vi "lijnvolgen.vi"() -> ()   [LabVIEW 2019]
uses:
  <vilib>/myRIO/Common/Instrument Driver Framework/Utilities/typedefs/Analog Scaling Constants.ctl
  <vilib>/myRIO/Common/Instrument Driver Framework/Utilities/typedefs/Analog Scaling Constants List.ctl
  <vilib>/myRIO/Common/Instrument Driver Framework/myRIO v1.0/AO/typedefs/AO Channels Enum.ctl
  <vilib>/myRIO/Common/Instrument Driver Framework/myRIO v1.0/AO/typedefs/AO Channels List.ctl
  <vilib>/myRIO/Common/Instrument Driver Framework/Utilities/typedefs/Generic FPGA Reference.ctl
  <vilib>/myRIO/Common/Instrument Driver Framework/Utilities/typedefs/myRIO v1.0 Reference.ctl
  <vilib>/myRIO/Common/Instrument Driver Framework/Utilities/typedefs/Hardware Version Enum.ctl
  <vilib>/myRIO/Common/Instrument Driver Framework/Utilities/typedefs/myRIO Generic Hardware Reference.ctl
  <vilib>/myRIO/Instrument Drivers/Onboard IO/AO/typedefs/AO Reference.ctl
  <vilib>/myRIO/Instrument Drivers/Onboard IO/AO/AO.lvlib
  <vilib>/myRIO/Instrument Drivers/Onboard IO/AO/vis/Write.vi
  <vilib>/userDefined/High Color/nirio_resource_hc.ctl
  <vilib>/myRIO/Common/Instrument Driver Framework/myRIO v1.0/AO/vis/myRIO v1.1 Open AO.vi
  <vilib>/myRIO/Instrument Drivers/Onboard IO/AO/vis/myRIO AO Open.xnode
  <vilib>/myRIO/Common/Instrument Driver Framework/Utilities/vis/Is FPGA Ref Available.vi
  <vilib>/myRIO/Express VI/Onboard IO/AO/AO Express VI.xnode
  <vilib>/myRIO/Common/Instrument Driver Framework/myRIO v1.0/AI/typedefs/AI Channels Enum.ctl
  <vilib>/myRIO/Common/Instrument Driver Framework/myRIO v1.0/AI/typedefs/AI Channels List.ctl
  <vilib>/myRIO/Instrument Drivers/Onboard IO/AI/typedefs/AI Reference.ctl
  <vilib>/myRIO/Instrument Drivers/Onboard IO/AI/AI.lvlib
  <vilib>/myRIO/Instrument Drivers/Onboard IO/AI/vis/Read.vi
  <vilib>/myRIO/Common/Instrument Driver Framework/myRIO v1.0/AI/vis/myRIO v1.1 Open AI.vi
  <vilib>/myRIO/Instrument Drivers/Onboard IO/AI/vis/myRIO AI Open.xnode
  <vilib>/myRIO/Express VI/Onboard IO/AI/AI Express VI.xnode
panel:
  in  "Boolean":bool
  out "Numeric 4":i32
  out "analoog":dbl[](array[numeric])
  out "Array 3":i32[](array[numeric])
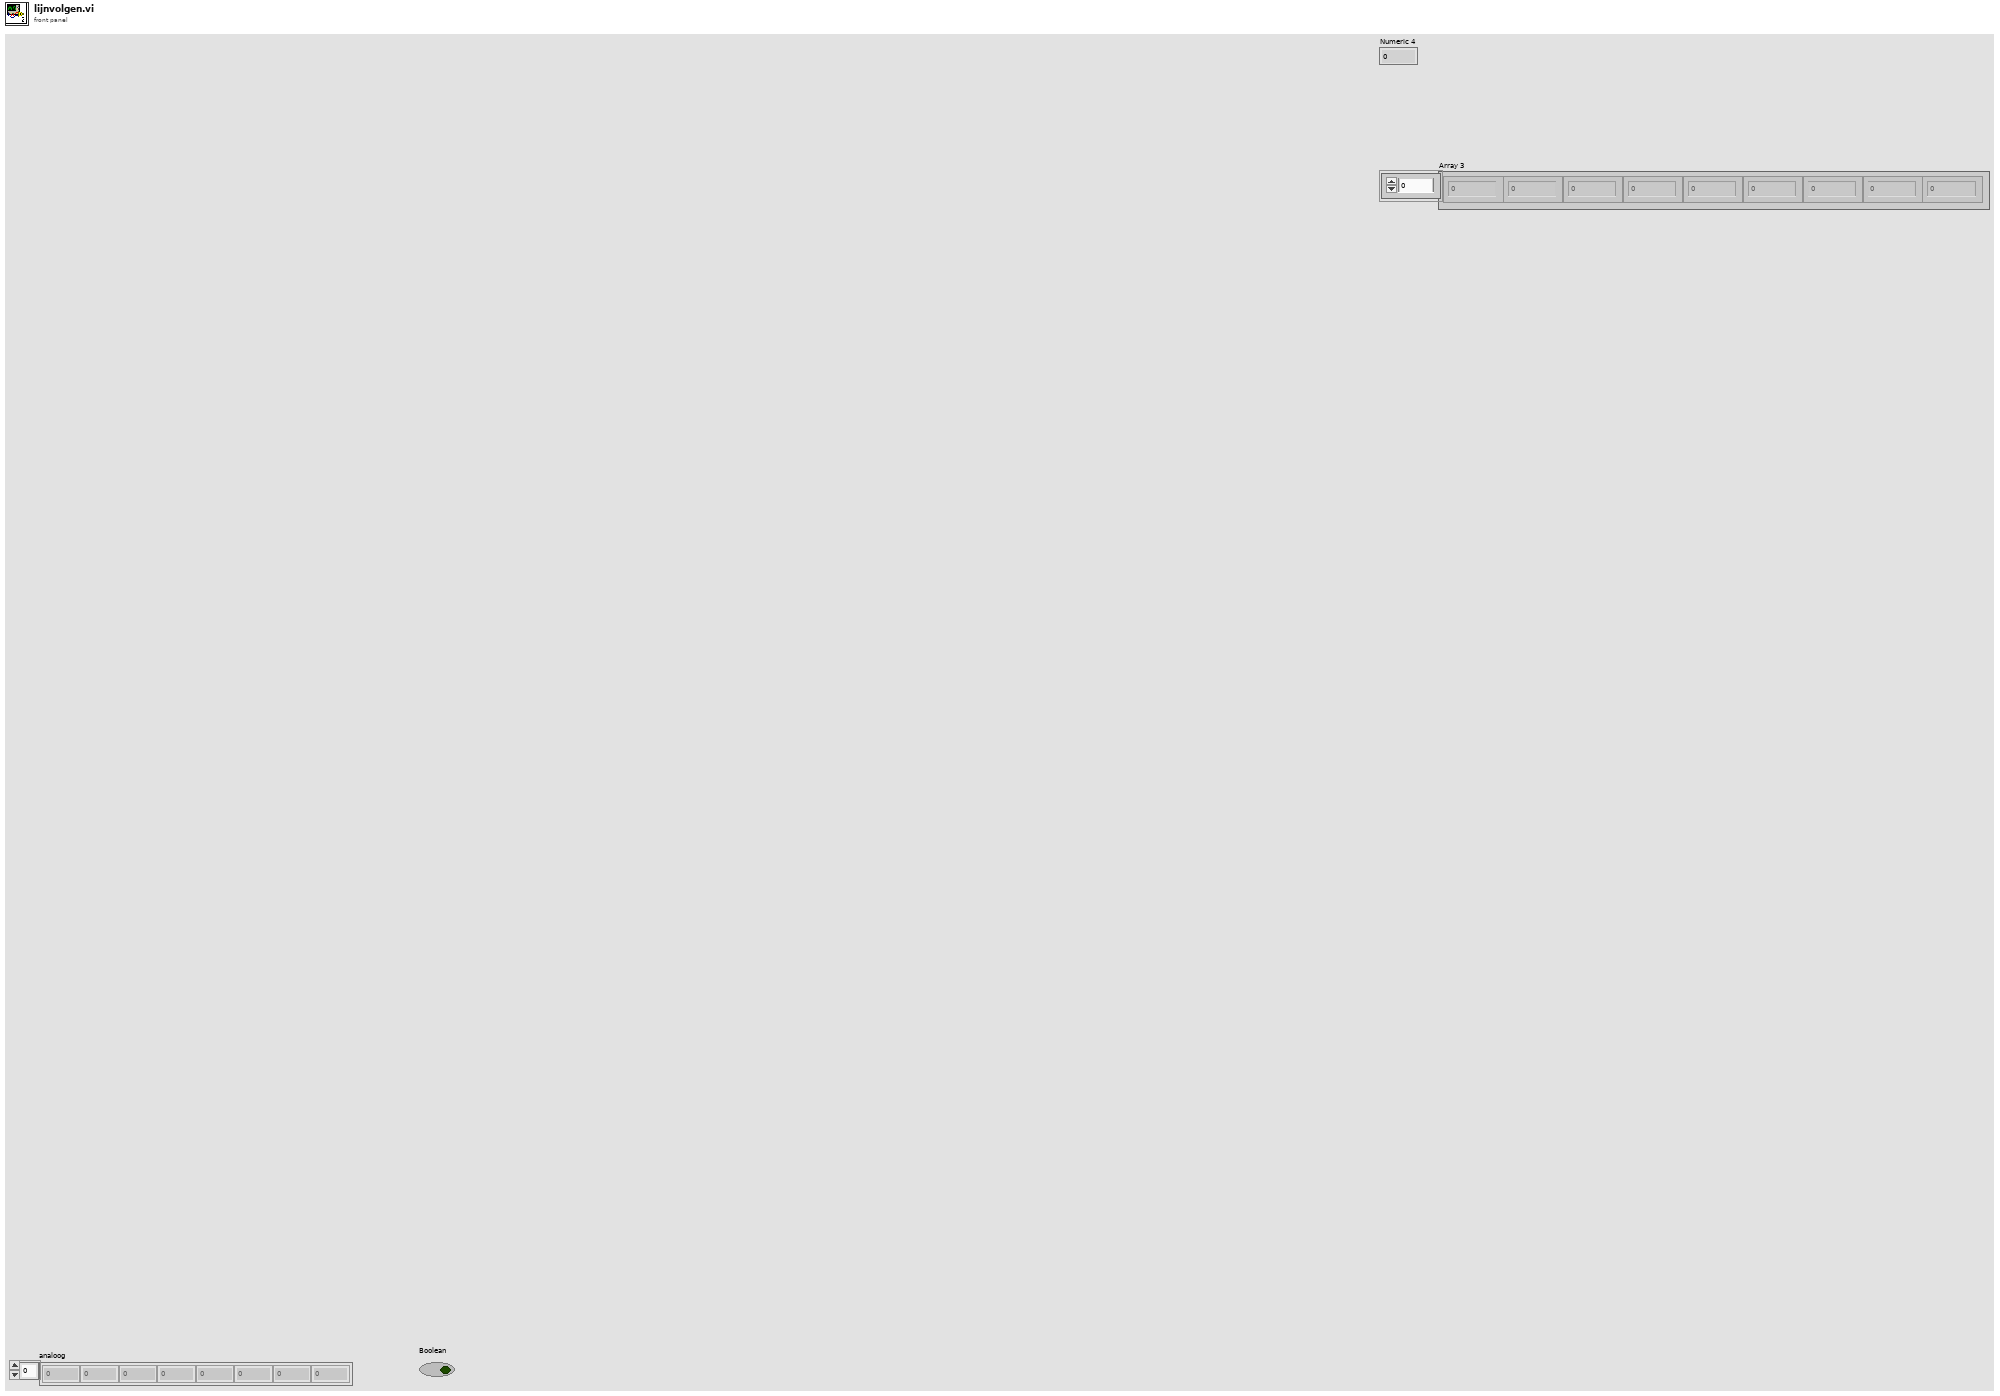
[diagram p1: front panel]
types:
  T1 = typedef "AO.lvlib/AO Reference.ctl" = cluster{"myRIO Reference":T2, "AO Channel List":T6, "AO Scaling Constant List":T8}
  T2 = typedef "myRIO Generic Hardware Reference.ctl" = cluster{"myRIO Model":T3, "myRIO Hardware Reference":T4}
  T3 = typedef "Hardware Version Enum.ctl" = enum16{"Unknown", "myRIO-1900", "myRIO-1950", "roboRIO", "NI ELVIS RIO CM", "ELVIS III"}
  T4 = typedef "myRIO v1.0 Reference.ctl" = cluster{"Generic FPGA Reference":T5, "Allow multiple opens":bool}
  T5 = typedef "Generic FPGA Reference.ctl" = refnum<k20>
  T6 = typedef "AO Channels List.ctl" = T7[]
  T7 = typedef "AO Channels Enum.ctl" = enum16{"Not Connected", "AudioOut/Left", "AudioOut/Right", "C/AO0", "C/AO1", "A/AO0", "A/AO1", "B/AO0", "B/AO1"}
  T8 = typedef "Analog Scaling Constants List.ctl" = T9[]
  T9 = typedef "Analog Scaling Constants.ctl" = cluster{"LSB Weight (Volts)":dbl, "Offset (Volts)":dbl, "Signed?":bool}
  T10 = typedef "nirio_resource_hc.ctl" = tag
  T11 = typedef "AI.lvlib/AI Reference.ctl" = cluster{"myRIO Reference":T2, "AI Channels List":T12, "AI Scaling Constants List":T8}
  T12 = typedef "AI Channels List.ctl" = T13[]
  T13 = typedef "AI Channels Enum.ctl" = enum16{"Not Connected", "AudioIn/Left", "AudioIn/Right", "C/AI0", "C/AI1", "A/AI0", "A/AI1", "A/AI2", "A/AI3", "A/AI4", "A/AI5", "A/AI6", "A/AI7", "B/AI0", "B/AI1", "B/AI2", "B/AI3", "B/AI4", "B/AI5", "B/AI6", "B/AI7", "AI/AI0", "AI/AI1", "AI/AI2", "AI/AI3", "A/AI0 (DIFF)", "A/AI1 (DIFF)", "A/AI2 (DIFF)", "A/AI3 (DIFF)", "B/AI0 (DIFF)", "B/AI1 (DIFF)", "B/AI2 (DIFF)", "B/AI3 (DIFF)"}
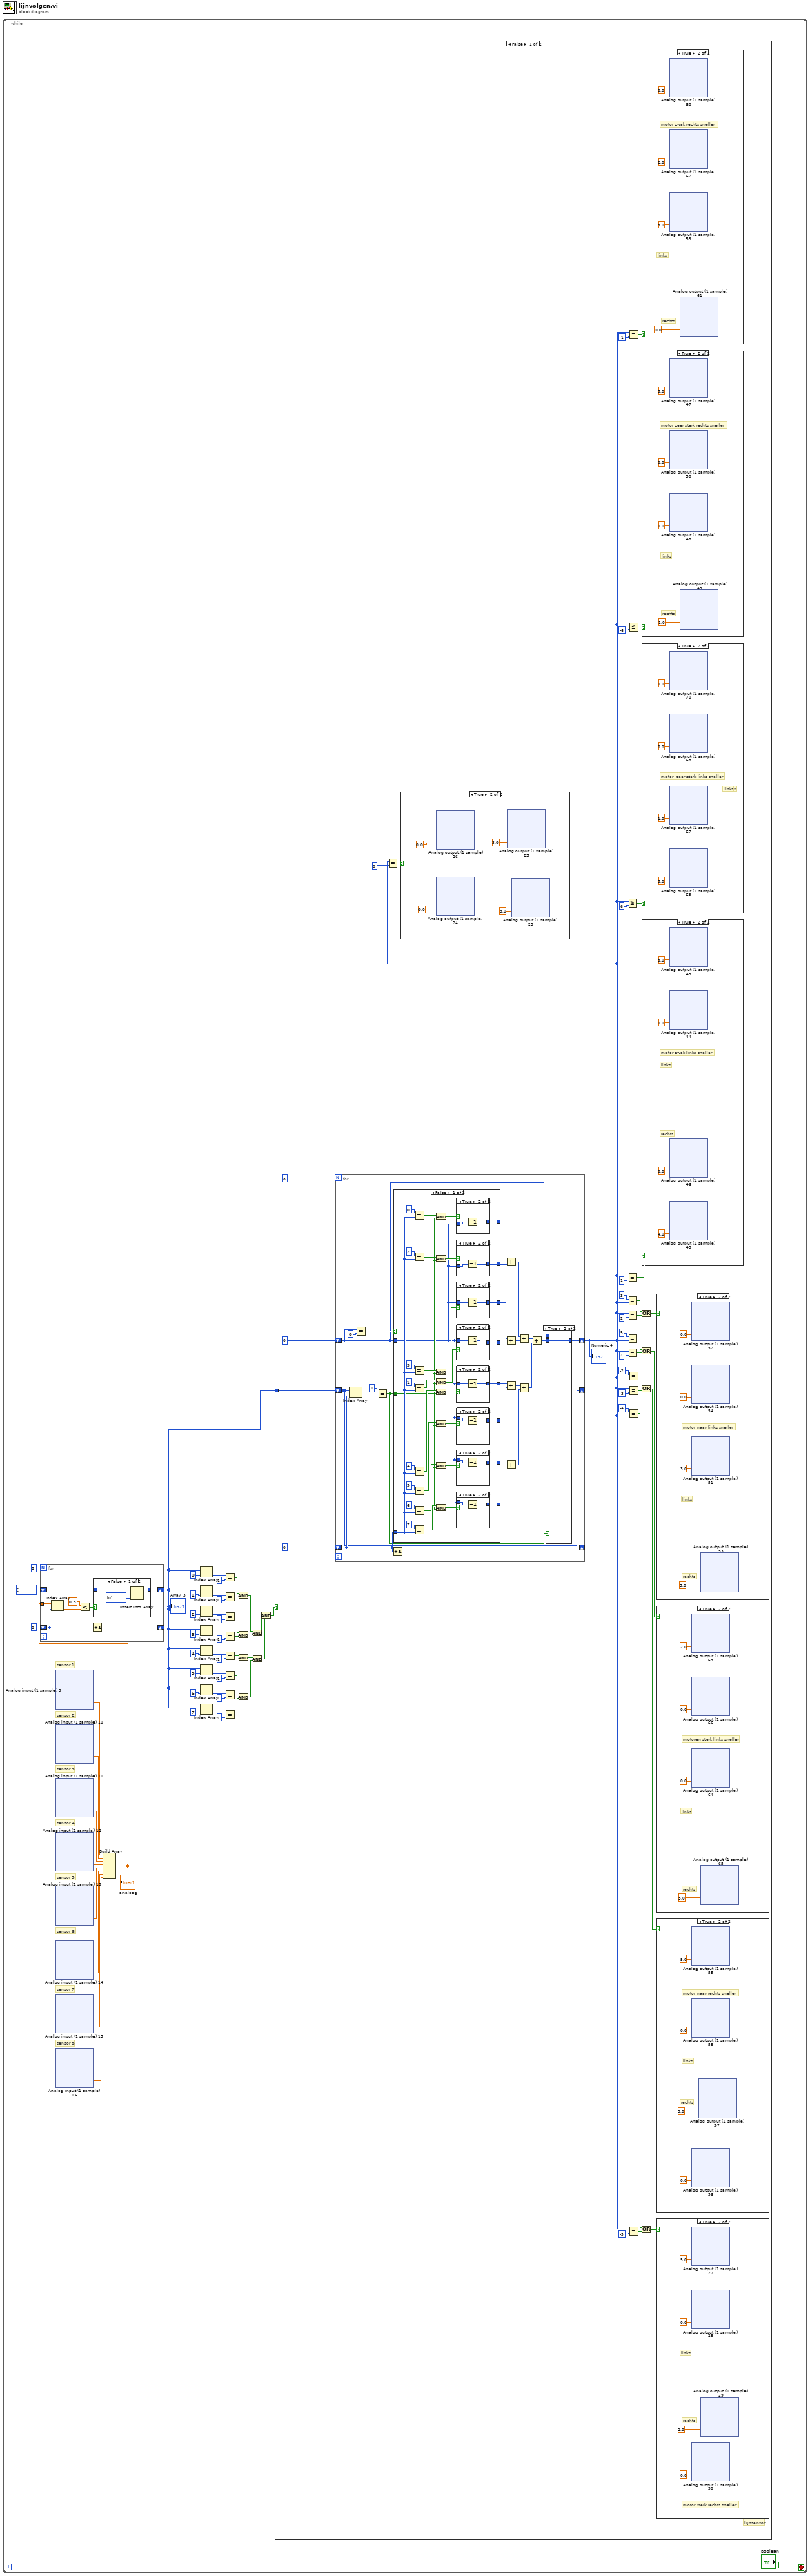
[diagram p0: block diagram]
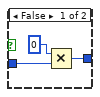
[diagram p12: hidden frame]
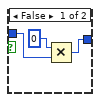
[diagram p13: hidden frame]
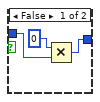
[diagram p14: hidden frame]
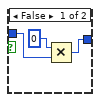
[diagram p15: hidden frame]
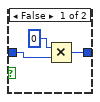
[diagram p16: hidden frame]
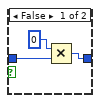
[diagram p17: hidden frame]
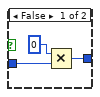
[diagram p18: hidden frame]
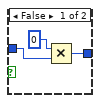
[diagram p19: hidden frame]
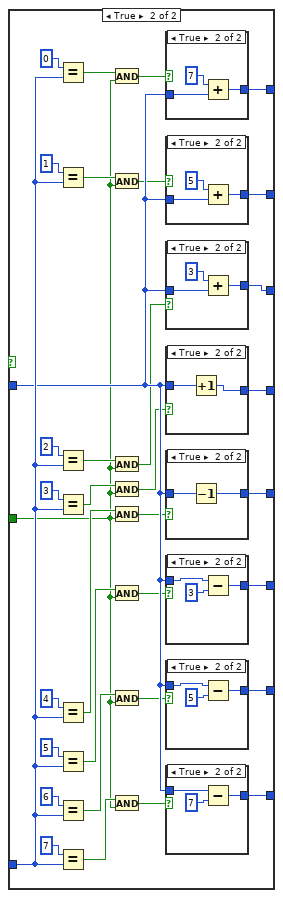
[diagram p20: hidden frame]
diagram:
  n1 = while {
    stop <- "Boolean" stop-if-true
    # "sensor 8"
    # "sensor 7"
    # "sensor 6"
    # "sensor 5"
    # "sensor 4"
    # "sensor 3"
    # "sensor 2"
    # "sensor 1"
    n2 = xnode "Analog input (1 sample) 9"() -> ("A/AI3 (Pin 9)"=w5:dbl)  [unwired: 1 in, 1 out]
    n3 = xnode "Analog input (1 sample) 10"() -> ("A/AI2 (Pin 7)"=w6:dbl)  [unwired: 1 in, 1 out]
    n4 = xnode "Analog input (1 sample) 11"() -> ("A/AI1 (Pin 5)"=w7:dbl)  [unwired: 1 in, 1 out]
    n5 = xnode "Analog input (1 sample) 12"() -> ("A/AI0 (Pin 3)"=w8:dbl)  [unwired: 1 in, 1 out]
    n6 = xnode "Analog input (1 sample) 13"() -> ("B/AI3 (Pin 9)"=w9:dbl)  [unwired: 1 in, 1 out]
    n7 = xnode "Analog input (1 sample) 14"() -> ("B/AI2 (Pin 7)"=w10:dbl)  [unwired: 1 in, 1 out]
    n8 = xnode "Analog input (1 sample) 15"() -> ("A/AI1 (Pin 5)"=w11:dbl)  [unwired: 1 in, 1 out]
    n9 = xnode "Analog input (1 sample) 16"() -> ("B/AI0 (Pin 3)"=w12:dbl)  [unwired: 1 in, 1 out]
    n10 = Build Array(w5, w6, w7, w8, w9, w10, w11, w12) -> (w4:dbl[])
    "analoog" <- w4
    n11 = for {
      N: 8 -> [_]
      shift-right: [w2094] -> w2
      shift-left: i32[] [] -> [w2095]
      shift-right: [w2091] -> _
      shift-left: 0 -> [w2090]
      tunnel: w4 -> [w2088]
      n12 = Index Array(array=w2088, index=w2090) -> (element=w2089:dbl)
      n13 = Less?(x=0.3, y=w2089) -> (x < y?=w2093:bool)
      n14 = Increment(x=w2090) -> (x+1=w2091:i32)
      n15 = case shown="False" w2093 {
        tunnel: w2095 -> [w2097 w2099]
        tunnel: [w2098 w2101] -> w2094
        frame False {
          n16 = Insert Into Array(array=w2097, new element=i32[] [0]) -> (w2098:i32[])  [unwired: 1 in]
        }
        frame True {
          n17 = Insert Into Array(array=w2099, new element=i32[] [1, 1]) -> (w2101:i32[])  [unwired: 1 in]
        }
      }
    }
    "Array 3" <- w2
    n18 = Index Array(array=w2, index=0) -> (element=w34:i32)
    n19 = Index Array(array=w2, index=1) -> (element=w13:i32)
    n20 = Index Array(array=w2, index=2) -> (element=w19:i32)
    n21 = Index Array(array=w2, index=3) -> (element=w16:i32)
    n22 = Index Array(array=w2, index=4) -> (element=w22:i32)
    n23 = Index Array(array=w2, index=5) -> (element=w25:i32)
    n24 = Index Array(array=w2, index=6) -> (element=w28:i32)
    n25 = Index Array(array=w2, index=7) -> (element=w31:i32)
    n26 = Equal?(x=w34, y=1) -> (x = y?=w37:bool)
    n27 = Equal?(x=w13, y=1) -> (x = y?=w38:bool)
    n28 = Equal?(x=w19, y=1) -> (x = y?=w39:bool)
    n29 = Equal?(x=w16, y=1) -> (x = y?=w40:bool)
    n30 = Equal?(x=w22, y=1) -> (x = y?=w41:bool)
    n31 = Equal?(x=w25, y=1) -> (x = y?=w42:bool)
    n32 = Equal?(x=w28, y=1) -> (x = y?=w43:bool)
    n33 = Equal?(x=w31, y=1) -> (x = y?=w44:bool)
    n34 = And(x=w37, y=w38) -> (x .and. y?=w45:bool)
    n35 = And(x=w39, y=w40) -> (x .and. y?=w46:bool)
    n36 = And(x=w41, y=w42) -> (x .and. y?=w47:bool)
    n37 = And(x=w43, y=w44) -> (x .and. y?=w48:bool)
    n38 = And(x=w45, y=w46) -> (x .and. y?=w49:bool)
    n39 = And(x=w47, y=w48) -> (x .and. y?=w50:bool)
    n40 = And(x=w49, y=w50) -> (x .and. y?=w3:bool)
    n41 = case shown="False" w3 {
      tunnel: w2 -> [w54 _]
      frame False {
        # "lijnsensor"
        n42 = for {
          N: 8 -> [_]
          shift-right: [w1467] -> _
          shift-left: 0 -> [w1481]
          shift-right: [w1459] -> w55
          shift-left: 0 -> [w1460]
          shift-right: [w1472] -> _
          shift-left: w54 -> [w1472]
          n43 = Index Array(array=w1472, index=w1481) -> (element=w1471:i32)
          n44 = Equal?(x=w1460, y=0) -> (x = y?=w1468:bool)
          n45 = Equal?(x=1, y=w1471) -> (x = y?=w1458:bool)
          n46 = Increment(x=w1481) -> (x+1=w1467:i32)
          n47 = case shown="False" w1468 {
            tunnel: w1481 -> [w1491 w1577]
            tunnel: [w1485 w1576] -> w1480
            tunnel: [w1492 w1575] -> w1479
            tunnel: [w1493 w1574] -> w1478
            tunnel: [w1494 w1573] -> w1477
            tunnel: w1460 -> [w1484 w1572]
            tunnel: w1458 -> [w1490 w1563]
            tunnel: [w1488 w1562] -> w1466
            tunnel: [w1489 w1561] -> w1465
            tunnel: [w1486 w1560] -> w1463
            tunnel: [w1487 w1559] -> w1462
            frame False {
              n48 = Equal?(x=0, y=w1491) -> (x = y?=w1511:bool)
              n49 = Equal?(x=2, y=w1491) -> (x = y?=w1517:bool)
              n50 = Equal?(x=3, y=w1491) -> (x = y?=w1518:bool)
              n51 = Equal?(x=1, y=w1491) -> (x = y?=w1503:bool)
              n52 = Equal?(x=4, y=w1491) -> (x = y?=w1515:bool)
              n53 = Equal?(x=5, y=w1491) -> (x = y?=w1516:bool)
              n54 = Equal?(x=6, y=w1491) -> (x = y?=w1514:bool)
              n55 = Equal?(x=7, y=w1491) -> (x = y?=w1513:bool)
              n56 = And(x=w1511, y=w1490) -> (x .and. y?=w1495:bool)
              n57 = And(x=w1517, y=w1490) -> (x .and. y?=w1497:bool)
              n58 = And(x=w1518, y=w1490) -> (x .and. y?=w1498:bool)
              n59 = And(x=w1503, y=w1490) -> (x .and. y?=w1496:bool)
              n60 = And(x=w1515, y=w1490) -> (x .and. y?=w1499:bool)
              n61 = And(x=w1516, y=w1490) -> (x .and. y?=w1500:bool)
              n62 = And(x=w1514, y=w1490) -> (x .and. y?=w1501:bool)
              n63 = And(x=w1513, y=w1490) -> (x .and. y?=w1502:bool)
              n64 = case shown="True" w1495 {
                tunnel: [w1520 w1523] -> w1489
                tunnel: w1484 -> [w1519 w1522]
                frame False {
                  n65 = Multiply(x=0, y=w1519) -> (x*y=w1520:i32)
                }
                frame True {
                  n66 = Decrement(x=w1522) -> (x-1=w1523:i32)
                }
              }
              n67 = case shown="True" w1497 {
                tunnel: [w1551 w1552] -> w1488
                tunnel: w1484 -> [w1550 w1553]
                frame False {
                  n68 = Multiply(x=0, y=w1550) -> (x*y=w1551:i32)
                }
                frame True {
                  n69 = Decrement(x=w1553) -> (x-1=w1552:i32)
                }
              }
              n70 = case shown="True" w1498 {
                tunnel: [w1545 w1548] -> w1487
                tunnel: w1484 -> [w1544 w1547]
                frame False {
                  n71 = Multiply(x=0, y=w1544) -> (x*y=w1545:i32)
                }
                frame True {
                  n72 = Decrement(x=w1547) -> (x-1=w1548:i32)
                }
              }
              n73 = case shown="True" w1496 {
                tunnel: [w1555 w1558] -> w1486
                tunnel: w1484 -> [w1554 w1557]
                frame False {
                  n74 = Multiply(x=0, y=w1554) -> (x*y=w1555:i32)
                }
                frame True {
                  n75 = Decrement(x=w1557) -> (x-1=w1558:i32)
                }
              }
              n76 = case shown="True" w1499 {
                tunnel: [w1540 w1543] -> w1485
                tunnel: w1484 -> [w1539 w1542]
                frame False {
                  n77 = Multiply(x=0, y=w1539) -> (x*y=w1540:i32)
                }
                frame True {
                  n78 = Decrement(x=w1542) -> (x-1=w1543:i32)
                }
              }
              n79 = case shown="True" w1500 {
                tunnel: [w1530 w1533] -> w1492
                tunnel: w1484 -> [w1529 w1532]
                frame False {
                  n80 = Multiply(x=0, y=w1529) -> (x*y=w1530:i32)
                }
                frame True {
                  n81 = Decrement(x=w1532) -> (x-1=w1533:i32)
                }
              }
              n82 = case shown="True" w1501 {
                tunnel: [w1535 w1538] -> w1493
                tunnel: w1484 -> [w1534 w1537]
                frame False {
                  n83 = Multiply(x=0, y=w1534) -> (x*y=w1535:i32)
                }
                frame True {
                  n84 = Decrement(x=w1537) -> (x-1=w1538:i32)
                }
              }
              n85 = case shown="True" w1502 {
                tunnel: [w1524 w1528] -> w1494
                tunnel: w1484 -> [w1525 w1527]
                frame False {
                  n86 = Multiply(x=0, y=w1525) -> (x*y=w1524:i32)
                }
                frame True {
                  n87 = Decrement(x=w1527) -> (x-1=w1528:i32)
                }
              }
            }
            frame True {
              n88 = Equal?(x=0, y=w1577) -> (x = y?=w1586:bool)
              n89 = Equal?(x=1, y=w1577) -> (x = y?=w1578:bool)
              n90 = Equal?(x=2, y=w1577) -> (x = y?=w1592:bool)
              n91 = Equal?(x=3, y=w1577) -> (x = y?=w1593:bool)
              n92 = Equal?(x=4, y=w1577) -> (x = y?=w1590:bool)
              n93 = Equal?(x=5, y=w1577) -> (x = y?=w1591:bool)
              n94 = Equal?(x=6, y=w1577) -> (x = y?=w1589:bool)
              n95 = Equal?(x=7, y=w1577) -> (x = y?=w1588:bool)
              n96 = And(x=w1586, y=w1563) -> (x .and. y?=w1564:bool)
              n97 = And(x=w1578, y=w1563) -> (x .and. y?=w1565:bool)
              n98 = And(x=w1592, y=w1563) -> (x .and. y?=w1566:bool)
              n99 = And(x=w1593, y=w1563) -> (x .and. y?=w1567:bool)
              n100 = And(x=w1590, y=w1563) -> (x .and. y?=w1568:bool)
              n101 = And(x=w1591, y=w1563) -> (x .and. y?=w1569:bool)
              n102 = And(x=w1589, y=w1563) -> (x .and. y?=w1570:bool)
              n103 = And(x=w1588, y=w1563) -> (x .and. y?=w1571:bool)
              n104 = case shown="True" w1564 {
                tunnel: w1572 -> [w1594 w1598]
                tunnel: [w1595 w1597] -> w1561
                frame False {
                  n105 = Multiply(x=0, y=w1594) -> (x*y=w1595:i32)
                }
                frame True {
                  n106 = Add(x=7, y=w1598) -> (x+y=w1597:i32)
                }
              }
              n107 = case shown="True" w1565 {
                tunnel: w1572 -> [w1634 w1637]
                tunnel: [w1635 w1638] -> w1562
                frame False {
                  n108 = Multiply(x=0, y=w1634) -> (x*y=w1635:i32)
                }
                frame True {
                  n109 = Add(x=5, y=w1637) -> (x+y=w1638:i32)
                }
              }
              n110 = case shown="True" w1566 {
                tunnel: w1572 -> [w1628 w1632]
                tunnel: [w1629 w1631] -> w1559
                frame False {
                  n111 = Multiply(x=0, y=w1628) -> (x*y=w1629:i32)
                }
                frame True {
                  n112 = Add(x=3, y=w1632) -> (x+y=w1631:i32)
                }
              }
              n113 = case shown="True" w1567 {
                tunnel: w1572 -> [w1624 w1627]
                tunnel: [w1623 w1626] -> w1560
                frame False {
                  n114 = Multiply(x=0, y=w1624) -> (x*y=w1623:i32)
                }
                frame True {
                  n115 = Increment(x=w1627) -> (x+1=w1626:i32)
                }
              }
              n116 = case shown="True" w1568 {
                tunnel: w1572 -> [w1618 w1622]
                tunnel: [w1619 w1621] -> w1576
                frame False {
                  n117 = Multiply(x=0, y=w1618) -> (x*y=w1619:i32)
                }
                frame True {
                  n118 = Decrement(x=w1622) -> (x-1=w1621:i32)
                }
              }
              n119 = case shown="True" w1569 {
                tunnel: w1572 -> [w1607 w1609]
                tunnel: [w1606 w1611] -> w1575
                frame False {
                  n120 = Multiply(x=0, y=w1607) -> (x*y=w1606:i32)
                }
                frame True {
                  n121 = Subtract(x=w1609, y=3) -> (x-y=w1611:i32)
                }
              }
              n122 = case shown="True" w1570 {
                tunnel: w1572 -> [w1613 w1615]
                tunnel: [w1612 w1616] -> w1574
                frame False {
                  n123 = Multiply(x=0, y=w1613) -> (x*y=w1612:i32)
                }
                frame True {
                  n124 = Subtract(x=w1615, y=5) -> (x-y=w1616:i32)
                }
              }
              n125 = case shown="True" w1571 {
                tunnel: w1572 -> [w1600 w1603]
                tunnel: [w1601 w1604] -> w1573
                frame False {
                  n126 = Multiply(x=0, y=w1600) -> (x*y=w1601:i32)
                }
                frame True {
                  n127 = Subtract(x=w1603, y=7) -> (x-y=w1604:i32)
                }
              }
            }
          }
          n128 = Add(x=w1465, y=w1466) -> (x+y=w1464:i32)
          n129 = Add(x=w1462, y=w1463) -> (x+y=w1461:i32)
          n130 = Add(x=w1480, y=w1479) -> (x+y=w1475:i32)
          n131 = Add(x=w1478, y=w1477) -> (x+y=w1476:i32)
          n132 = Add(x=w1464, y=w1461) -> (x+y=w1474:i32)
          n133 = Add(x=w1475, y=w1476) -> (x+y=w1473:i32)
          n134 = Add(x=w1474, y=w1473) -> (x+y=w1457:i32)
          n135 = case shown="True" w1458 {
            tunnel: w1460 -> [w1482 _]
            tunnel: [w1482 w1483] -> w1459
            tunnel: w1457 -> [_ w1483]
            frame False {
            }
            frame True {
            }
          }
        }
        "Numeric 4" <- w55
        n136 = Equal?(x=w55, y=0) -> (x = y?=w57:bool)
        n137 = case shown="True" w57 {
          frame False {
          }
          frame True {
            n138 = xnode "Analog output (1 sample) 24"("B/AO0 (Pin 2)"=0.0) -> ()  [unwired: 1 in, 1 out]
            n139 = xnode "Analog output (1 sample) 26"("A/AO0 (Pin 2)"=0.0) -> ()  [unwired: 1 in, 1 out]
            n140 = xnode "Analog output (1 sample) 25"("A/AO1 (Pin 4)"=3.0) -> ()  [unwired: 1 in, 1 out]
            n141 = xnode "Analog output (1 sample) 23"("B/AO1 (Pin 4)"=3.0) -> ()  [unwired: 1 in, 1 out]
          }
        }
        n142 = Greater Or Equal?(x=w55, y=6) -> (x >= y?=w83:bool)
        n143 = Equal?(x=w55, y=1) -> (x = y?=w84:bool)
        n144 = Equal?(x=3, y=w55) -> (x = y?=w74:bool)
        n145 = Equal?(x=w55, y=2) -> (x = y?=w75:bool)
        n146 = Equal?(x=5, y=w55) -> (x = y?=w78:bool)
        n147 = Equal?(x=w55, y=4) -> (x = y?=w79:bool)
        n148 = Equal?(x=w55, y=-1) -> (x = y?=w62:bool)
        n149 = Less Or Equal?(x=w55, y=-6) -> (x <= y?=w60:bool)
        n150 = Equal?(x=-2, y=w55) -> (x = y?=w68:bool)
        n151 = Equal?(x=w55, y=-3) -> (x = y?=w69:bool)
        n152 = Equal?(x=-4, y=w55) -> (x = y?=w64:bool)
        n153 = Equal?(x=w55, y=-5) -> (x = y?=w65:bool)
        n154 = Or(x=w74, y=w75) -> (x .or. y?=w72:bool)
        n155 = Or(x=w78, y=w79) -> (x .or. y?=w80:bool)
        n156 = Or(x=w68, y=w69) -> (x .or. y?=w61:bool)
        n157 = Or(x=w64, y=w65) -> (x .or. y?=w58:bool)
        n158 = case shown="True" w62 {
          frame False {
          }
          frame True {
            # "rechts"
            # "links"
            # "motor zwak rechts sneller"
            n159 = xnode "Analog output (1 sample) 60"("B/AO1 (Pin 4)"=0.0) -> ()  [unwired: 1 in, 1 out]
            n160 = xnode "Analog output (1 sample) 62"("A/AO0 (Pin 2)"=2.0) -> ()  [unwired: 1 in, 1 out]
            n161 = xnode "Analog output (1 sample) 59"("B/AO0 (Pin 2)"=5.0) -> ()  [unwired: 1 in, 1 out]
            n162 = xnode "Analog output (1 sample) 61"("A/AO1 (Pin 4)"=0.0) -> ()  [unwired: 1 in, 1 out]
          }
        }
        n163 = case shown="True" w60 {
          frame False {
          }
          frame True {
            # "rechts"
            # "links"
            # "motor zeer sterk rechts sneller"
            n164 = xnode "Analog output (1 sample) 47"("B/AO1 (Pin 4)"=5.0) -> ()  [unwired: 1 in, 1 out]
            n165 = xnode "Analog output (1 sample) 50"("A/AO0 (Pin 2)"=0.0) -> ()  [unwired: 1 in, 1 out]
            n166 = xnode "Analog output (1 sample) 48"("B/AO0 (Pin 2)"=0.0) -> ()  [unwired: 1 in, 1 out]
            n167 = xnode "Analog output (1 sample) 49"("A/AO1 (Pin 4)"=1.0) -> ()  [unwired: 1 in, 1 out]
          }
        }
        n168 = case shown="True" w83 {
          frame False {
          }
          frame True {
            # "rechts"
            # "links"
            # "motor  zeer sterk links sneller"
            n169 = xnode "Analog output (1 sample) 70"("A/AO0 (Pin 2)"=0.0) -> ()  [unwired: 1 in, 1 out]
            n170 = xnode "Analog output (1 sample) 68"("B/AO0 (Pin 2)"=0.0) -> ()  [unwired: 1 in, 1 out]
            n171 = xnode "Analog output (1 sample) 67"("B/AO1 (Pin 4)"=1.0) -> ()  [unwired: 1 in, 1 out]
            n172 = xnode "Analog output (1 sample) 69"("A/AO1 (Pin 4)"=5.0) -> ()  [unwired: 1 in, 1 out]
          }
        }
        n173 = case shown="True" w84 {
          frame False {
          }
          frame True {
            # "rechts"
            # "links"
            # "motor zwak links sneller"
            n174 = xnode "Analog output (1 sample) 45"("A/AO1 (Pin 4)"=5.0) -> ()  [unwired: 1 in, 1 out]
            n175 = xnode "Analog output (1 sample) 44"("B/AO0 (Pin 2)"=0.0) -> ()  [unwired: 1 in, 1 out]
            n176 = xnode "Analog output (1 sample) 46"("A/AO0 (Pin 2)"=0.0) -> ()  [unwired: 1 in, 1 out]
            n177 = xnode "Analog output (1 sample) 43"("B/AO1 (Pin 4)"=4.0) -> ()  [unwired: 1 in, 1 out]
          }
        }
        n178 = case shown="True" w72 {
          frame False {
          }
          frame True {
            # "rechts"
            # "links"
            # "motor naar links sneller"
            n179 = xnode "Analog output (1 sample) 52"("B/AO0 (Pin 2)"=0.0) -> ()  [unwired: 1 in, 1 out]
            n180 = xnode "Analog output (1 sample) 54"("A/AO0 (Pin 2)"=0.0) -> ()  [unwired: 1 in, 1 out]
            n181 = xnode "Analog output (1 sample) 51"("B/AO1 (Pin 4)"=3.0) -> ()  [unwired: 1 in, 1 out]
            n182 = xnode "Analog output (1 sample) 53"("A/AO1 (Pin 4)"=5.0) -> ()  [unwired: 1 in, 1 out]
          }
        }
        n183 = case shown="True" w80 {
          frame False {
          }
          frame True {
            # "rechts"
            # "links"
            # "motoren sterk links sneller"
            n184 = xnode "Analog output (1 sample) 63"("B/AO1 (Pin 4)"=2.0) -> ()  [unwired: 1 in, 1 out]
            n185 = xnode "Analog output (1 sample) 66"("A/AO0 (Pin 2)"=0.0) -> ()  [unwired: 1 in, 1 out]
            n186 = xnode "Analog output (1 sample) 64"("B/AO0 (Pin 2)"=0.0) -> ()  [unwired: 1 in, 1 out]
            n187 = xnode "Analog output (1 sample) 65"("A/AO1 (Pin 4)"=5.0) -> ()  [unwired: 1 in, 1 out]
          }
        }
        n188 = case shown="True" w61 {
          frame False {
          }
          frame True {
            # "rechts"
            # "links"
            # "motor naar rechts sneller"
            n189 = xnode "Analog output (1 sample) 55"("B/AO1 (Pin 4)"=5.0) -> ()  [unwired: 1 in, 1 out]
            n190 = xnode "Analog output (1 sample) 58"("A/AO0 (Pin 2)"=0.0) -> ()  [unwired: 1 in, 1 out]
            n191 = xnode "Analog output (1 sample) 56"("B/AO0 (Pin 2)"=0.0) -> ()  [unwired: 1 in, 1 out]
            n192 = xnode "Analog output (1 sample) 57"("A/AO1 (Pin 4)"=3.0) -> ()  [unwired: 1 in, 1 out]
          }
        }
        n193 = case shown="True" w58 {
          frame False {
          }
          frame True {
            # "rechts"
            # "links"
            # "motor sterk rechts sneller"
            n194 = xnode "Analog output (1 sample) 27"("B/AO1 (Pin 4)"=5.0) -> ()  [unwired: 1 in, 1 out]
            n195 = xnode "Analog output (1 sample) 28"("B/AO0 (Pin 2)"=0.0) -> ()  [unwired: 1 in, 1 out]
            n196 = xnode "Analog output (1 sample) 30"("A/AO0 (Pin 2)"=0.0) -> ()  [unwired: 1 in, 1 out]
            n197 = xnode "Analog output (1 sample) 29"("A/AO1 (Pin 4)"=2.0) -> ()  [unwired: 1 in, 1 out]
          }
        }
      }
      frame True {
        n198 = xnode "Analog output (1 sample)"("A/AO0 (Pin 2)"=0) -> ()  [unwired: 1 in, 1 out]
        n199 = xnode "Analog output (1 sample) 3"("B/AO0 (Pin 2)"=0) -> ()  [unwired: 1 in, 1 out]
        n200 = xnode "Analog output (1 sample) 2"("A/AO1 (Pin 4)"=0) -> ()  [unwired: 1 in, 1 out]
        n201 = xnode "Analog output (1 sample) 4"("B/AO1 (Pin 4)"=0) -> ()  [unwired: 1 in, 1 out]
      }
    }
  }
